vi "from string.vi"(8 "error in":errorcluster, 9 "data":string, 10 "version":string, 11 "SystemLin Tag Module configuration in":refnum<class "SystemLink File configuration.lvclass">) -> (0 "error out":errorcluster, 3 "SystemLin Tag Module configuration out":refnum<class "SystemLink File configuration.lvclass">)   [LabVIEW 2015, in "SystemLink File configuration.lvclass"]
doc: "Provides an interface for loading a module configuration from a file or other serialized data source. It is recommended that all children of this class store data in two sets--data required for its own initialization, and any data required for parent initialization--and that each implementation uses the <b>Call Parent Method</b> primitive to de-serialize parent information. As a result, it is expected that every module configuration class calls <b>component configuration.lvclass:From String.vi</b>."
uses:
  SystemLink File configuration.lvclass
  Connection Configuration.ctl
  Connection Type.ctl
  <vilib>/NI/Tag Bus Module Framework/channel/TBM channel.lvclass
  SystemLink File configuration.lvclass/SystemLink File configuration.ctl
  <vilib>/NI/Tag Bus Module Framework/module configuration/TBM module configuration.lvclass
  <vilib>/NI/Configuration Framework/serializable configuration/NISE_CEF_serializable configuration.lvclass
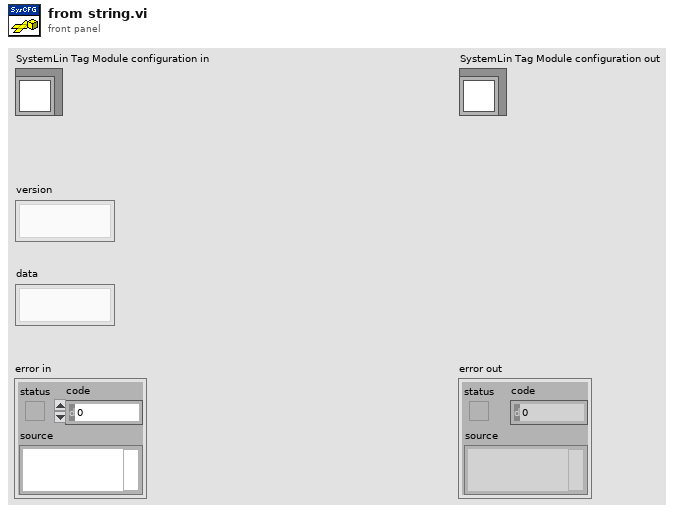
[diagram p1: front panel]
types:
  T1 = typedef "SystemLink File configuration.lvclass/Connection Configuration.ctl" = cluster{"Connection Type":T2, "AMQP":cluster{"Configuration ID":string}, "HTTP":cluster{"Verify Server?":bool, "Server URL":string, "CA Certificate File":string, "User Info":cluster{"Username":string, "Password":string}, "API Key":string}}
  T2 = typedef "SystemLink File configuration.lvclass/Connection Type.ctl" = enum16{"AMQP", "HTTP", "API Key (SystemLink Cloud)"}
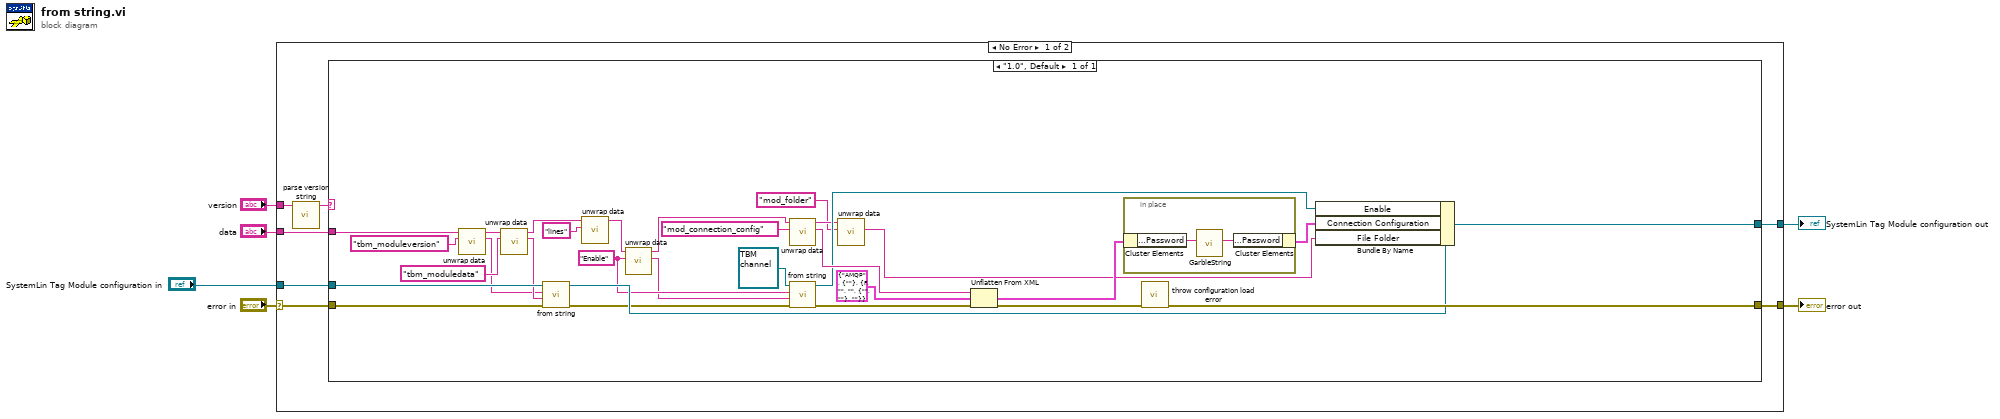
[diagram p0: block diagram]
diagram:
  n1 = case shown="No Error" "error in" {
    selector: "error in" -> [w7 w47]
    tunnel: "data" -> [w13 _]
    tunnel: "SystemLin Tag Module configuration in" -> [w12 w46]
    tunnel: [w11 w46] -> w5
    tunnel: [w10 w47] -> w4
    tunnel: "version" -> [w9 _]
    frame No Error {
      n2 = call <vilib>:"parse version string.vi"("full version"=w9) -> ("major.minor version"=w8:string)  [unwired: 7 in, 3 out]
      n3 = case shown="\"1.0\", Default" w8 {
        tunnel: w13 -> [w40]
        tunnel: w7 -> [w39]
        tunnel: w12 -> [w43]
        tunnel: [w31] -> w11
        tunnel: [w42] -> w10
        frame "1.0", Default {
          w15 = "Enable" ("identifier")
          n4 = call <vilib>:"unwrap data.vi"("identifier"="tbm_moduleversion" ("additional identifier"), "data to unwrap"=w40) -> ("unwrapped data"=w35:string, "remaining string"=w41:string)  [unwired: 8 in]
          n5 = call <vilib>:"unwrap data.vi"("identifier"="tbm_moduledata" ("additional identifier"), "data to unwrap"=w41) -> ("unwrapped data"=w37:string, "remaining string"=w34:string)  [unwired: 8 in]
          n6 = call-parent "from string.vi"("error in"=w39, "data"=w37, "version"=w35, "module configuration in"=w43) -> ("error out"=w29:errorcluster, "module configuration out"=w32:refnum<class "SystemLink File configuration.lvclass">)  [unwired: 6 in]
          n7 = call <vilib>:"unwrap data.vi"("identifier"="lines" ("additional identifier"), "data to unwrap"=w34) -> ("remaining string"=w30:string)  [unwired: 8 in, 1 out]
          n8 = call <vilib>:"unwrap data.vi"("identifier"=w15, "data to unwrap"=w30) -> ("unwrapped data"=w14:string, "remaining string"=w28:string)  [unwired: 8 in]
          n9 = call <vilib>:"unwrap data.vi"("identifier"="mod_connection_config", "data to unwrap"=w28) -> ("unwrapped data"=w26:string, "remaining string"=w18:string)  [unwired: 8 in]
          n10 = call-dynamic "from string.vi"("error in"=w29, "channel data"=w14, "identifier"=w15, "channel in"=refnum<class "TBM channel.lvclass"> refnum) -> ("error out"=w25:errorcluster, "channel out"=w19:refnum<class "TBM channel.lvclass">)  [unwired: 6 in]
          n11 = call <vilib>:"unwrap data.vi"("identifier"="mod_folder", "data to unwrap"=w18) -> ("unwrapped data"=w16:string)  [unwired: 8 in, 1 out]
          n12 = Unflatten From XML(xml string=w26, type=T1 {"Connection Type"=enum."AMQP", "AMQP"={"Configuration ID"=""}, "HTTP"={"Verify Server?"=FALSE, "Server URL"="", "CA Certificate File"="", "User Info"={"Username"="", "Password"=""}, "API Key"=""}} ("anything"), error in (no error)=w25) -> (value=w21:T1, error out=w24:errorcluster)
          n13 = in-place {
            n14 = in-place-cluster #1(w21) -> ("HTTP.User Info.Password"=w45:string)
            n15 = call "GarbleString.vi"("String In"=w45) -> ("String Out"=w44:string)  [unwired: 10 in]
            n16 = in-place-cluster #1("HTTP.User Info.Password"=w44) -> (w22:T1)
          }
          n17 = call <vilib>:"throw configuration load error.vi"("error in"=w24) -> ("error out"=w42:errorcluster)  [unwired: 10 in]
          n18 = Bundle By Name(cluster=w32, "Enable"=w19, "Connection Configuration"=w22, "File Folder"=w16) -> (w31:refnum<class "SystemLink File configuration.lvclass">)
        }
      }
    }
    frame Error {
    }
  }
  "error out" <- w4
  "SystemLin Tag Module configuration out" <- w5
